vi "Main.vi"() -> ()   [LabVIEW 2018]
uses:
  StateENUM.ctl
  1d93126f-b57a-4b2e-a5e1-2b10a66ae46b.vi
  <vilib>/Instr/_visa.llb/VISA Configure Serial Port (Instr).vi
panel:
  in  "Check Center":bool
  out "Step":i32
  in  "Increase Step":bool
  in  "Decrease Step":bool
  out "Center":i32
  out "LoopCount":i32
  in  "Jitter Up":bool
  in  "Jitter Down":bool
  out "Command Buffer":string
  in  "stop":bool
  out "Current Time":timestamp format="%<%I:%M:%S %p | %m/%d/%y>T"
  in  "VISA resource name":refnum<visa-resource-name>="COM9"
  in  "Up Button":bool
  in  "Down Button":bool
  # "Manual\nAdjustment"
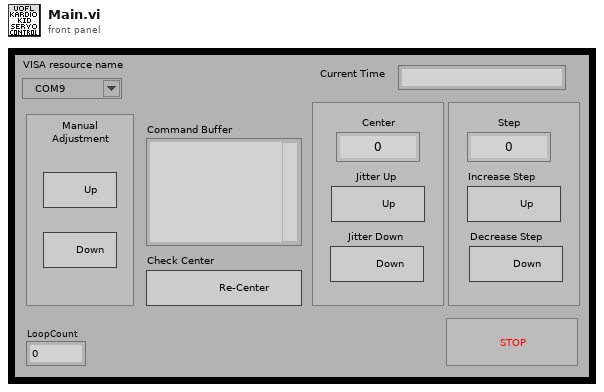
[diagram p1: front panel]
types:
  T1 = typedef "StateENUM.ctl" = enum16{"Init", "Idle", "MoveUp", "MoveDown", "JitterUp", "JitterDown", "IncreaseStep", "DecreaseStep", "CheckCenter", "ReadSerial", "ScanData", "Shutdown"}
  T2 = typedef "MoveCommands.ctl" = cluster{"MoveUp":string, "MoveDown":string, "JitterUp":string, "JitterDown":string, "IncStep":string, "DecStep":string, "ChkCenter":string}
  T3 = cluster{"VISA resource name out":refnum<visa-resource-name>, "error out":errorcluster, "State":T1, "Stop":bool, "Buffer":string, "Center":i32, "Step":i32, "SerialIncoming?":bool, "MoveCommands":T2}
  T4 = cluster{"Command Buffer":refnum<vi>, "Jitter Up":refnum<vi>, "Jitter Down":refnum<vi>, "Increase Step":refnum<vi>, "Decrease Step":refnum<vi>}
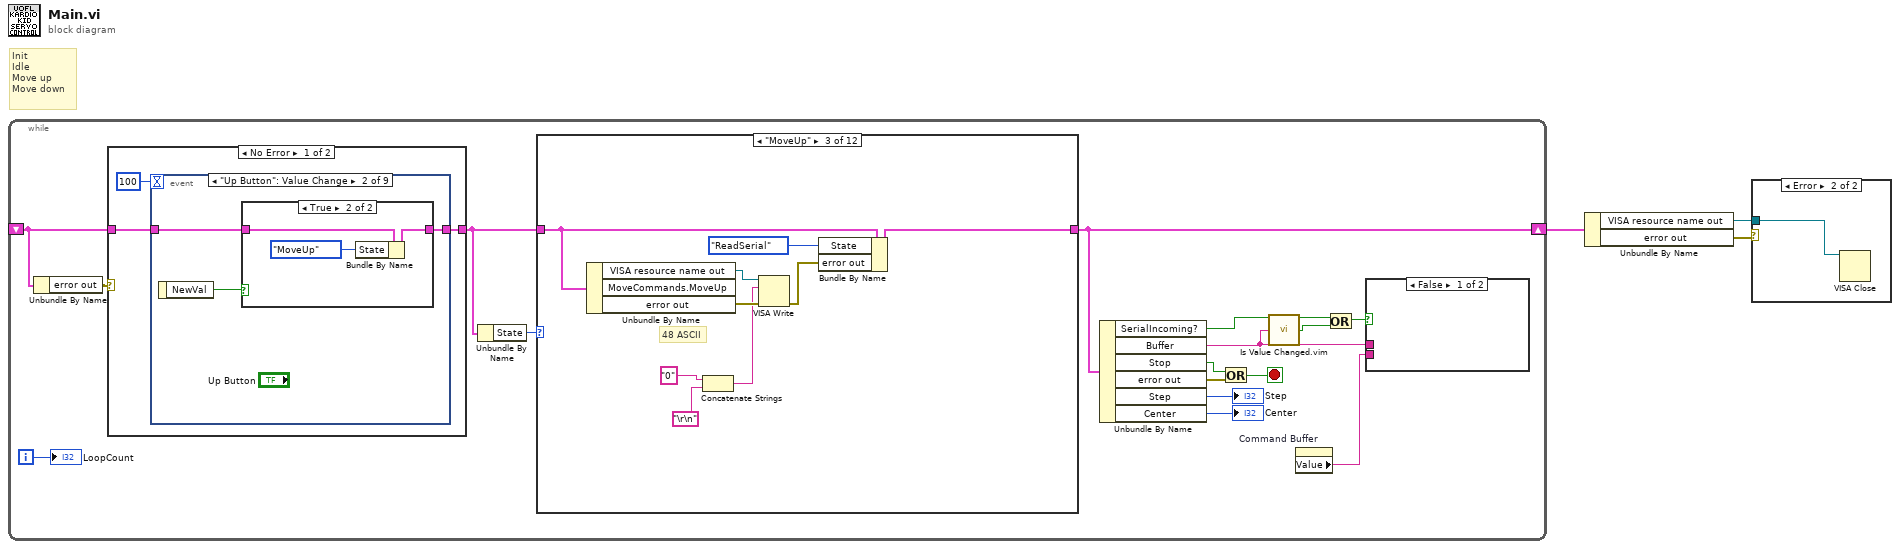
[diagram p0: block diagram]
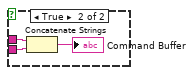
[diagram p3: hidden frame]
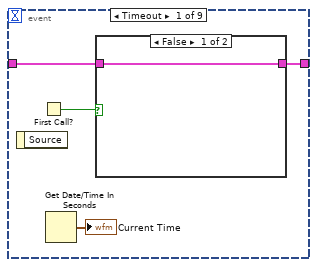
[diagram p4: hidden frame]
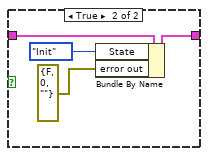
[diagram p5: hidden frame]
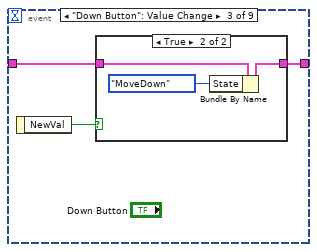
[diagram p7: hidden frame]
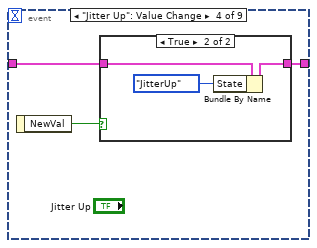
[diagram p9: hidden frame]
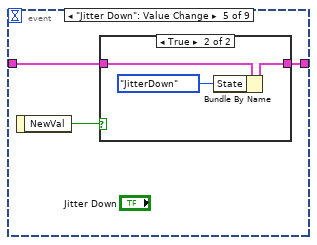
[diagram p11: hidden frame]
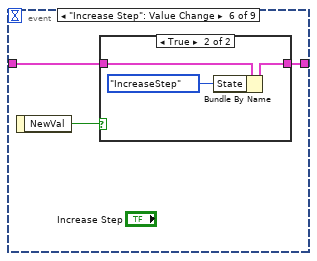
[diagram p13: hidden frame]
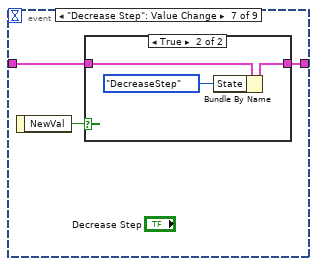
[diagram p15: hidden frame]
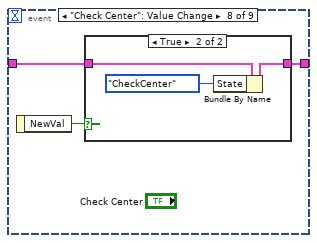
[diagram p17: hidden frame]
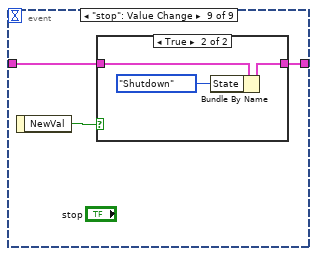
[diagram p19: hidden frame]
diagram:
  # "Init\nIdle\nMove up\nMove down"
  n1 = while {
    shift-right: [w17] -> w3
    shift-left: _ -> [w16]
    i -> [w14]
    stop <- w13 stop-if-true
    n2 = Unbundle By Name(w16) -> ("error out"=w15:errorcluster)
    n3 = case shown="No Error" w15 {
      tunnel: w16 -> [w24 w97]
      tunnel: [w23 w93] -> w18
      frame No Error {
        n4 = event shown="[1] \"Up Button\": Value Change" {
          selector: _ -> [_ _ _ _ _ _ _ _ _]
          dyn-events: _ -> [_ _ _ _ _ _ _ _ _]
          timeout: 100 -> [_ _ _ _ _ _ _ _ _]
          tunnel: w24 -> [w26 w37 w43 w51 w58 w65 w72 w79 w85]
          tunnel: [w27 w35 w42 w49 w56 w63 w70 w77 w84] -> w23
          event Timeout {
            n5 = event-data() -> ()  [unwired: 1 in, 1 out]
            n6 = First Call?() -> (First Call?: T/F=w28:bool)
            n7 = Get Date/Time In Seconds() -> (seconds since 1Jan1904=→"Current Time":timestamp)
            n8 = case shown="False" w28 {
              tunnel: [w30 w33] -> w27
              tunnel: w26 -> [w30 w34]
              frame False {
              }
              frame True {
                n9 = Bundle By Name(cluster=w34, "State"=StateENUM."Init", "error out"=errorcluster {"status"=FALSE, "code"=0, "source"=""}) -> (w33:T3)
              }
            }
          }
          event "Up Button": Value Change {
            n10 = event-data() -> ("NewVal"=w36:bool)  [unwired: 1 in]
            n11 = case shown="True" w36 {
              tunnel: w37 -> [w38 w41]
              tunnel: [w38 w40] -> w35
              frame False {
              }
              frame True {
                n12 = Bundle By Name(cluster=w41, "State"=StateENUM."MoveUp") -> (w40:T3)
              }
            }
          }
          event "Down Button": Value Change {
            n13 = event-data() -> ("NewVal"=w44:bool)  [unwired: 1 in]
            n14 = case shown="True" w44 {
              tunnel: w43 -> [w45 w48]
              tunnel: [w45 w47] -> w42
              frame False {
              }
              frame True {
                n15 = Bundle By Name(cluster=w48, "State"=StateENUM."MoveDown") -> (w47:T3)
              }
            }
          }
          event "Jitter Up": Value Change {
            n16 = event-data() -> ("NewVal"=w50:bool)  [unwired: 1 in]
            n17 = case shown="True" w50 {
              tunnel: w51 -> [w52 w55]
              tunnel: [w52 w54] -> w49
              frame False {
              }
              frame True {
                n18 = Bundle By Name(cluster=w55, "State"=StateENUM."JitterUp") -> (w54:T3)
              }
            }
          }
          event "Jitter Down": Value Change {
            n19 = event-data() -> ("NewVal"=w57:bool)  [unwired: 1 in]
            n20 = case shown="True" w57 {
              tunnel: w58 -> [w59 w62]
              tunnel: [w59 w61] -> w56
              frame False {
              }
              frame True {
                n21 = Bundle By Name(cluster=w62, "State"=StateENUM."JitterDown") -> (w61:T3)
              }
            }
          }
          event "Increase Step": Value Change {
            n22 = event-data() -> ("NewVal"=w64:bool)  [unwired: 1 in]
            n23 = case shown="True" w64 {
              tunnel: w65 -> [w66 w69]
              tunnel: [w66 w68] -> w63
              frame False {
              }
              frame True {
                n24 = Bundle By Name(cluster=w69, "State"=StateENUM."IncreaseStep") -> (w68:T3)
              }
            }
          }
          event "Decrease Step": Value Change {
            n25 = event-data() -> ("NewVal"=w71:bool)  [unwired: 1 in]
            n26 = case shown="True" w71 {
              tunnel: w72 -> [w73 w76]
              tunnel: [w73 w75] -> w70
              frame False {
              }
              frame True {
                n27 = Bundle By Name(cluster=w76, "State"=StateENUM."DecreaseStep") -> (w75:T3)
              }
            }
          }
          event "Check Center": Value Change {
            n28 = event-data() -> ("NewVal"=w78:bool)  [unwired: 1 in]
            n29 = case shown="True" w78 {
              tunnel: w79 -> [w80 w83]
              tunnel: [w80 w82] -> w77
              frame False {
              }
              frame True {
                n30 = Bundle By Name(cluster=w83, "State"=StateENUM."CheckCenter") -> (w82:T3)
              }
            }
          }
          event "stop": Value Change {
            n31 = event-data() -> ("NewVal"=w86:bool)  [unwired: 1 in]
            n32 = case shown="True" w86 {
              tunnel: w85 -> [w87 w90]
              tunnel: [w87 w89] -> w84
              frame False {
              }
              frame True {
                n33 = Bundle By Name(cluster=w90, "State"=StateENUM."Shutdown") -> (w89:T3)
              }
            }
          }
        }
      }
      frame Error {
        n34 = Unbundle By Name(w97) -> ("error out"=w96:errorcluster)
        n35 = call <vilib>:"Simple Error Handler.vi"("error in (no error)"=w96) -> ("code out"=w94:i32, "error out"=w95:errorcluster)  [unwired: 4 in, 3 out]
        n36 = call <vilib>:"Clear Errors.vi"("error in (no error)"=w95, "specific error code to clear (0: all)"=w94) -> ("error out"=w92:errorcluster)  [unwired: 4 in, 1 out]
        n37 = Bundle By Name(cluster=w97, "error out"=w92, "State"=StateENUM."Shutdown") -> (w93:T3)
      }
    }
    n38 = Unbundle By Name(w18) -> ("State"=w19:T1)
    n39 = case shown="\"MoveUp\"" w19 {
      tunnel: [w111 w127 w137 w144 w152 w161 w168 w175 w182 w197 w214 w245] -> w17
      tunnel: w18 -> [_ w129 w138 w145 w154 w163 w170 w177 w184 w198 w215 w247]
      frame "Init", Default {
        w99 = FALSE  # SerialIncoming?
        w101 = 50  # Step
        w102 = 1500  # Center
        w104 = ""  # Buffer
        w109 = FALSE  # Stop
        w110 = StateENUM."Idle"  # State
        n40 = disable-structure shown="Enabled" {
          frame Disabled {
            n41 = control-ref of="Jitter Up"() -> (w114:refnum<vi>)
            n42 = control-ref of="Jitter Down"() -> (w115:refnum<vi>)
            n43 = control-ref of="Increase Step"() -> (w116:refnum<vi>)
            n44 = control-ref of="Decrease Step"() -> (w117:refnum<vi>)
            n45 = control-ref of="Command Buffer"() -> (w113:refnum<vi>)
            n46 = Bundle("Command Buffer"=w113, "Jitter Up"=w114, "Jitter Down"=w115, "Increase Step"=w116, "Decrease Step"=w117) -> (w112:T4)  [unwired: 1 in]
            n47 = call "InitPostions (SubVI).vi"("ControlCluster"=w112) -> ()  [unwired: 11 in]
          }
          frame Enabled {
          }
        }
        n48 = call-poly "VISA Configure Serial Port"("VISA resource name"="VISA resource name") -> ("VISA resource name out"=w107:refnum<visa-resource-name>, "error out"=w106:errorcluster)  [unwired: 13 in]
        n49 = VISA Flush I/O Buffer(VISA resource name=w107, error in (no error)=w106) -> (VISA resource name out=w100:refnum<visa-resource-name>, error out=w105:errorcluster)  [unwired: 1 in]
        n50 = call "MoveCommands (SubVI).vi"() -> ("MoveCommands"=w98:T2)  [unwired: 11 in]
        n51 = Wait (ms)(milliseconds to wait=u32 5) -> ()  [unwired: 1 out]
        n52 = Bundle("VISA resource name out"=w100, "error out"=w105, "State"=w110, "Stop"=w109, "Buffer"=w104, "Center"=w102, "Step"=w101, "SerialIncoming?"=w99, "MoveCommands"=w98) -> (w111:T3)  [unwired: 1 in]
      }
      frame "Idle" {
        n53 = Unbundle By Name(w129) -> ("State"=w120:T1, "VISA resource name out"=w126:refnum<visa-resource-name>, "error out"=w125:errorcluster)
        n54 = Wait (ms)(milliseconds to wait=u32 5) -> ()  [unwired: 1 out]
        n55 = property class="Instr"(reference=w126, error in=w125) -> (error out=w124:errorcluster, "Serial Settings:Number of Bytes at Serial Port"=w122:u32)  [unwired: 1 out]
        n56 = Greater Than 0?(x=w122) -> (x > 0?=w119:bool)
        n57 = Select(t=StateENUM."ReadSerial" ("State"), s=w119, f=w120) -> (s? t:f=w123:T1)
        n58 = Bundle By Name(cluster=w129, "State"=w123, "error out"=w124, "SerialIncoming?"=FALSE) -> (w127:T3)
      }
      frame "MoveUp" {
        # "48 ASCII"
        n59 = Unbundle By Name(w138) -> ("VISA resource name out"=w133:refnum<visa-resource-name>, "error out"=w134:errorcluster)  [unwired: 1 out]
        n60 = Concatenate Strings("0", "\r\n") -> (w130:string)
        n61 = VISA Write(VISA resource name=w133, write buffer=w130, error in (no error)=w134) -> (error out=w135:errorcluster)  [unwired: 2 out]
        n62 = Bundle By Name(cluster=w138, "State"=StateENUM."ReadSerial", "error out"=w135) -> (w137:T3)
      }
      frame "MoveDown" {
        # "49 ASCII"
        n63 = Unbundle By Name(w145) -> ("VISA resource name out"=w140:refnum<visa-resource-name>, "MoveCommands.MoveDown"=w139:string, "error out"=w141:errorcluster)
        n64 = VISA Write(VISA resource name=w140, write buffer=w139, error in (no error)=w141) -> (error out=w142:errorcluster)  [unwired: 2 out]
        n65 = Bundle By Name(cluster=w145, "State"=StateENUM."ReadSerial", "error out"=w142) -> (w144:T3)
      }
      frame "JitterUp" {
        n66 = Unbundle By Name(w154) -> ("Center"=w149:i32, "VISA resource name out"=w153:refnum<visa-resource-name>, "MoveCommands.JitterUp"=w146:string, "error out"=w147:errorcluster)
        n67 = Increment(x=w149) -> (x+1=w148:i32)
        n68 = VISA Write(VISA resource name=w153, write buffer=w146, error in (no error)=w147) -> (error out=w150:errorcluster)  [unwired: 2 out]
        n69 = Bundle By Name(cluster=w154, "State"=StateENUM."ReadSerial", "Center"=w148, "error out"=w150) -> (w152:T3)
      }
      frame "JitterDown" {
        n70 = Unbundle By Name(w163) -> ("Center"=w158:i32, "VISA resource name out"=w162:refnum<visa-resource-name>, "MoveCommands.JitterDown"=w155:string, "error out"=w156:errorcluster)
        n71 = Decrement(x=w158) -> (x-1=w157:i32)
        n72 = VISA Write(VISA resource name=w162, write buffer=w155, error in (no error)=w156) -> (error out=w159:errorcluster)  [unwired: 2 out]
        n73 = Bundle By Name(cluster=w163, "State"=StateENUM."ReadSerial", "Center"=w157, "error out"=w159) -> (w161:T3)
      }
      frame "IncreaseStep" {
        n74 = Unbundle By Name(w170) -> ("VISA resource name out"=w169:refnum<visa-resource-name>, "MoveCommands.IncStep"=w164:string, "error out"=w165:errorcluster)
        n75 = VISA Write(VISA resource name=w169, write buffer=w164, error in (no error)=w165) -> (error out=w166:errorcluster)  [unwired: 2 out]
        n76 = Bundle By Name(cluster=w170, "State"=StateENUM."ReadSerial", "error out"=w166) -> (w168:T3)
      }
      frame "DecreaseStep" {
        n77 = Unbundle By Name(w177) -> ("VISA resource name out"=w176:refnum<visa-resource-name>, "MoveCommands.DecStep"=w172:string, "error out"=w171:errorcluster)
        n78 = VISA Write(VISA resource name=w176, write buffer=w172, error in (no error)=w171) -> (error out=w173:errorcluster)  [unwired: 2 out]
        n79 = Bundle By Name(cluster=w177, "State"=StateENUM."ReadSerial", "error out"=w173) -> (w175:T3)
      }
      frame "CheckCenter" {
        n80 = Unbundle By Name(w184) -> ("VISA resource name out"=w183:refnum<visa-resource-name>, "MoveCommands.ChkCenter"=w178:string, "error out"=w179:errorcluster)
        n81 = VISA Write(VISA resource name=w183, write buffer=w178, error in (no error)=w179) -> (error out=w180:errorcluster)  [unwired: 2 out]
        n82 = Bundle By Name(cluster=w184, "State"=StateENUM."ReadSerial", "error out"=w180) -> (w182:T3)
      }
      frame "ReadSerial" {
        n83 = Unbundle By Name(w198) -> ("VISA resource name out"=w193:refnum<visa-resource-name>, "error out"=w188:errorcluster, "Buffer"=w187:string)
        n84 = Wait (ms)(milliseconds to wait=u32 5) -> ()  [unwired: 1 out]
        n85 = property class="Instr"(reference=w193, error in=w188) -> (reference out=w190:refnum<visa-resource-name>, error out=w189:errorcluster, "Serial Settings:Number of Bytes at Serial Port"=w191:u32)
        n86 = Greater Than 0?(x=w191) -> (x > 0?=w192:bool)
        n87 = case shown="True" w192 {
          selector: w192 -> [w200 w204]
          tunnel: [w201 w209] -> w195
          tunnel: [w202 w208] -> w194
          tunnel: w189 -> [w202 w207]
          tunnel: w190 -> [_ w206]
          tunnel: w191 -> [_ w205]
          tunnel: w187 -> [w201 _]
          tunnel: [w200 w204] -> w186
          tunnel: [StateENUM."Idle" ("State") StateENUM."ScanData" ("State")] -> w185
          frame False {
          }
          frame True {
            n88 = VISA Read(VISA resource name=w206, byte count=w205, error in (no error)=w207) -> (read buffer=w209:string, error out=w208:errorcluster)  [unwired: 2 out]
          }
        }
        n89 = Bundle By Name(cluster=w198, "State"=w185, "SerialIncoming?"=w186, "Buffer"=w195, "error out"=w194) -> (w197:T3)
      }
      frame "ScanData" {
        n90 = Unbundle By Name(w215) -> ("Buffer"=w216:string)
        n91 = call <vilib>:"Space Constant.vi"() -> ("String"=w211:string)
        n92 = Match Pattern(string=w216, regular expression=w211) -> (before substring=w210:string, after substring=w212:string)  [unwired: 1 in, 2 out]
        n93 = case shown="\"Center\", \"Stop\"" w210 {
          tunnel: "is " -> [_ w230 w240]
          tunnel: w212 -> [_ w229 w239]
          tunnel: w215 -> [w220 w225 w235]
          tunnel: [w219 w223 w233] -> w214
          frame Default {
            n94 = Bundle By Name(cluster=w220, "State"=StateENUM."Idle", "SerialIncoming?"=FALSE) -> (w219:T3)
          }
          frame "Center", "Stop" {
            n95 = Match Pattern(string=w229, regular expression=w230) -> (after substring=w227:string)  [unwired: 1 in, 3 out]
            n96 = Match Pattern(string=w227, regular expression="\r\n") -> (before substring=w226:string)  [unwired: 1 in, 3 out]
            n97 = Decimal String To Number(string=w226) -> (number=w224:i32)  [unwired: 2 in, 1 out]
            n98 = Bundle By Name(cluster=w225, "SerialIncoming?"=FALSE, "State"=StateENUM."Idle", "Center"=w224) -> (w223:T3)
          }
          frame "Step" {
            n99 = Match Pattern(string=w239, regular expression=w240) -> (after substring=w237:string)  [unwired: 1 in, 3 out]
            n100 = Match Pattern(string=w237, regular expression="\r\n") -> (before substring=w236:string)  [unwired: 1 in, 3 out]
            n101 = Decimal String To Number(string=w236) -> (number=w234:i32)  [unwired: 2 in, 1 out]
            n102 = Bundle By Name(cluster=w235, "SerialIncoming?"=FALSE, "State"=StateENUM."Idle", "Step"=w234) -> (w233:T3)
          }
        }
      }
      frame "Shutdown" {
        n103 = Unbundle By Name(w247) -> ("VISA resource name out"=w246:refnum<visa-resource-name>, "error out"=w241:errorcluster)
        n104 = VISA Close(VISA resource name=w246, error in (no error)=w241) -> (error out=w242:errorcluster)
        n105 = Bundle By Name(cluster=w247, "Stop"=TRUE, "State"=StateENUM."Shutdown", "error out"=w242) -> (w245:T3)
      }
    }
    n106 = Unbundle By Name(w17) -> ("SerialIncoming?"=w6:bool, "Buffer"=w10:string, "Stop"=w12:bool, "error out"=w11:errorcluster, "Step"=→"Step":i32, "Center"=→"Center":i32)
    n107 = Or(x=w12, y=w11) -> (x .or. y?=w13:bool)
    n108 = call "Is Value Changed.vim"("value"=w10) -> ("changed or first call?"=w8:bool)
    n109 = property on="Command Buffer" class="Str"() -> ("Value"=w9:string)  [unwired: 2 in, 2 out]
    n110 = Or(x=w6, y=w8) -> (x .or. y?=w7:bool)
    n111 = case shown="False" w7 {
      tunnel: w10 -> [_ w22]
      tunnel: w9 -> [_ w21]
      frame False {
      }
      frame True {
        n112 = Concatenate Strings(w22, w21) -> (→"Command Buffer":string)
      }
    }
    "LoopCount" <- w14
  }
  n113 = Unbundle By Name(w3) -> ("VISA resource name out"=w1:refnum<visa-resource-name>, "error out"=w2:errorcluster)
  n114 = case shown="Error" w2 {
    tunnel: w1 -> [_ w248]
    frame No Error {
    }
    frame Error {
      n115 = VISA Close(VISA resource name=w248) -> ()  [unwired: 1 in, 1 out]
    }
  }
